vi "unflatten.vi"(8 "error in (no error)":errorcluster, 10 "PID Loop String":string, 11 "Identifier":string) -> (0 "error out":errorcluster, 3 "PID Loop out":refnum<class "PID Loop.lvclass">)   [LabVIEW 2014, in "PID Loop.lvclass"]
uses:
  PID Loop.lvclass
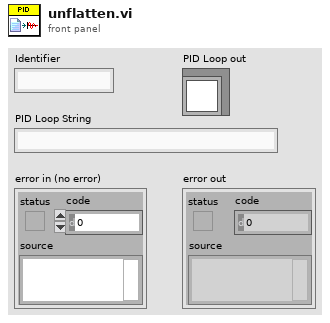
[diagram p1: front panel]
types:
  T1 = typedef "PID Loop.lvclass/PID Range.ctl" = cluster{"output high":dbl, "output low":dbl}
  T2 = typedef "PID Loop.lvclass/PID Parameters.ctl" = cluster{"Setpoint Tag":string, "Process Variable Tag":string, "Output Tag":string}
  T3 = typedef "PID Loop.lvclass/PID Gains.ctl" = cluster{"proportional gain (Kc)":dbl, "integral time (Ti, min)":dbl, "derivative time (Td, min)":dbl}
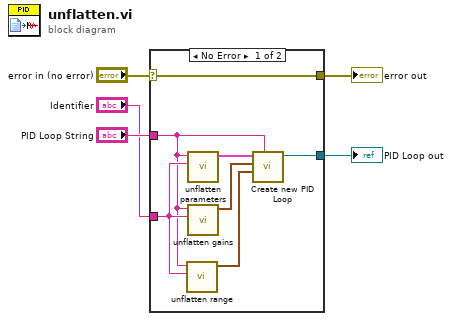
[diagram p0: block diagram]
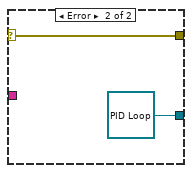
[diagram p2: hidden frame]
diagram:
  n1 = case shown="No Error" "error in (no error)" {
    selector: "error in (no error)" -> [w12 w14]
    tunnel: [w12 w14] -> w4
    tunnel: [w11 refnum<class "PID Loop.lvclass"> refnum ("PID Loop out")] -> w3
    tunnel: "PID Loop String" -> [w8 _]
    tunnel: "Identifier" -> [w9 _]
    frame No Error {
      n2 = call "unflatten range.vi"("Identifier"=w9, "Data to Unwrap"=w8) -> ("output range"=w7:T1)  [unwired: 9 in]
      n3 = call "unflatten parameters.vi"("Identifier"=w9, "Data to Unwrap"=w8) -> ("PID Parameters"=w6:T2)  [unwired: 9 in]
      n4 = call "unflatten gains.vi"("Identifier"=w9, "Data to Unwrap"=w8) -> ("PID gains"=w10:T3)  [unwired: 9 in]
      n5 = call "Create new PID Loop.vi"("ID"=w8, "output range"=w7, "PID gains"=w10, "PID Parameters"=w6) -> ("PID Loop out"=w11:refnum<class "PID Loop.lvclass">)  [unwired: 6 in, 1 out]
    }
    frame Error {
    }
  }
  "error out" <- w4
  "PID Loop out" <- w3
